vi "Controller whole.vi"() -> ()   [LabVIEW 2017]
uses:
  Global 1.vi
panel:
  in  "back to inipos":bool
  out "From Python":string
  in  "stop":bool
  in  "LA Auto/cal":bool
  in  "Shot - Act/pas":bool
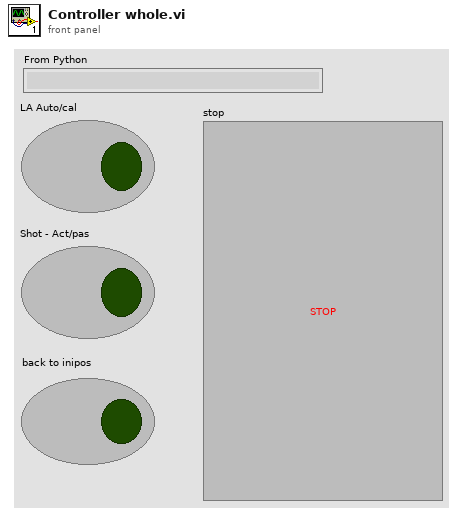
[diagram p1: front panel]
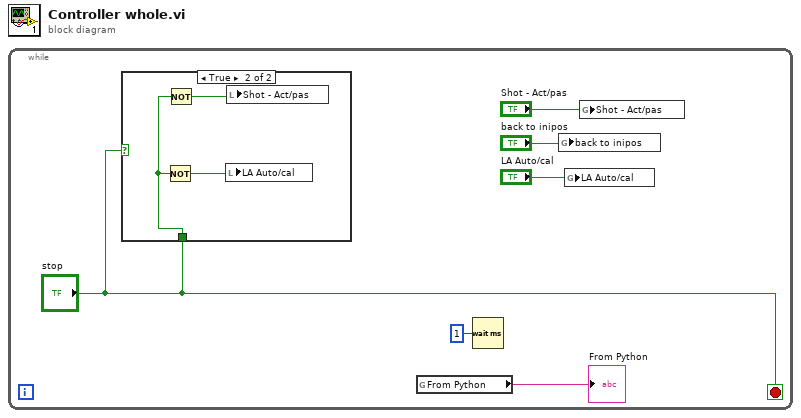
[diagram p0: block diagram]
diagram:
  n1 = while {
    stop <- "stop" stop-if-true
    n2 = case shown="True" "stop" {
      tunnel: "stop" -> [_ w9]
      frame False {
      }
      frame True {
        n3 = Not(x=w9) -> (.not. x?=w7:bool)
        n4 = Not(x=w9) -> (.not. x?=w8:bool)
        n5 = local write "LA Auto/cal"(w7) -> ()
        n6 = local write "Shot - Act/pas"(w8) -> ()
      }
    }
    n7 = global read "Global 1.vi" "From Python"() -> (→"From Python":string)
    n8 = Wait (ms)(milliseconds to wait=u32 1) -> ()  [unwired: 1 out]
    n9 = global write "Global 1.vi" "back to inipos"("back to inipos") -> ()
    n10 = global write "Global 1.vi" "LA Auto/cal"("LA Auto/cal") -> ()
    n11 = global write "Global 1.vi" "Shot - Act/pas"("Shot - Act/pas") -> ()
  }
